vi "Measurement UI.vi"() -> ()   [LabVIEW 2021, in "ADC_ACMeasurement.lvlib"]
uses:
  adc_acMeasurement.lvlib
panel:
  in  "MeasGraphs":T1(tab)
  out "FreqDomainGraph":cluster{"x0":dbl, "dx":dbl, "magnitude":dbl[]}(graph) caption="AC"
  out "TimeDomainGraph":waveform(dbl)(graph) caption="AC"
  out "ENOB":dbl
  out "SFDR":dbl
  out "SINAD":dbl
  out "THD":dbl
  out "SNR":dbl
  out "Calculated amplitude":dbl
  out "Calculated frequency":dbl
  out "Channel name":string
  out "Time domain":dbl[](array[numeric])
  out "dt":dbl
  out "t0":dbl
  out "Spectrum":dbl[](array[numeric])
  out "df":dbl
  out "f0":dbl
  in  "Analog source resource name":string
  in  "Digital capture resource name":string
  out "MeasTable":string[][](table)
  in  "Digital capture":string="Digital capture"
  in  "Analog source":string="Analog source"
  in  "MeasSettingsOptions":i32(listbox)
  in  "MeasSettings":bool
  in  "Digital capture samples":u32=800000 caption="NUMBER OF SAMPLES"
  in  "Input channel":i32 caption="INPUT CHANNEL" min=0 max=100 step=1
  in  "Full scale range":dbl=10.0 caption="FULL SCALE RANGE" format="%#_6pV"
  in  "Digital capture sample rate":dbl=800000.0 caption="SAMPLE RATE" format="%#_6pS/s"
  in  "Amplitude":dbl=-1.0 caption="AMPLITUDE" format="%#_6pdB"
  in  "Frequency":dbl=1000.0 caption="FREQUENCY" format="%#_6pHz"
  in  "DSGResourceName":tag caption="RESOURCE NAME"
  in  "DPIResourceName":refnum<k15> caption="RESOURCE NAME"
  in  "ADCparameters":string="ADC parameters"
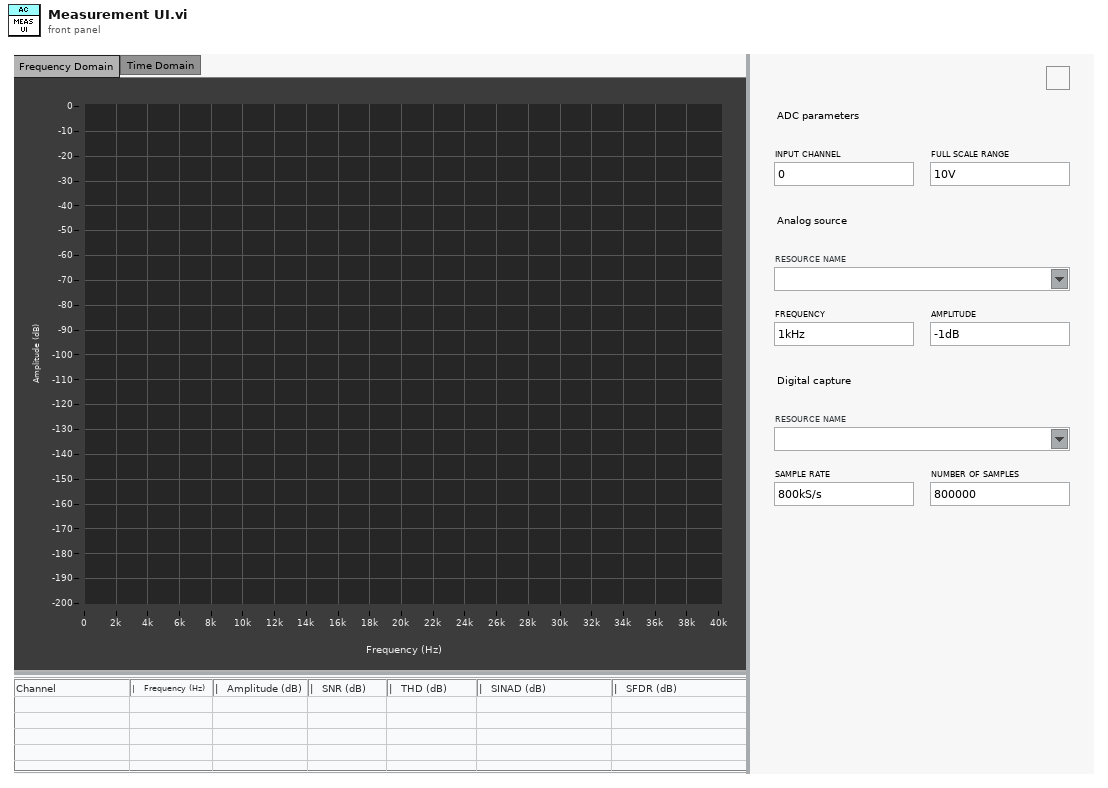
[diagram p1: front panel]
types:
  T1 = enum32{"Frequency Domain", "Time Domain", "Hidden Controls"}
  T2 = enum16{"open", "replace", "create", "open or create", "replace or create", "replace or create with confirmation"}
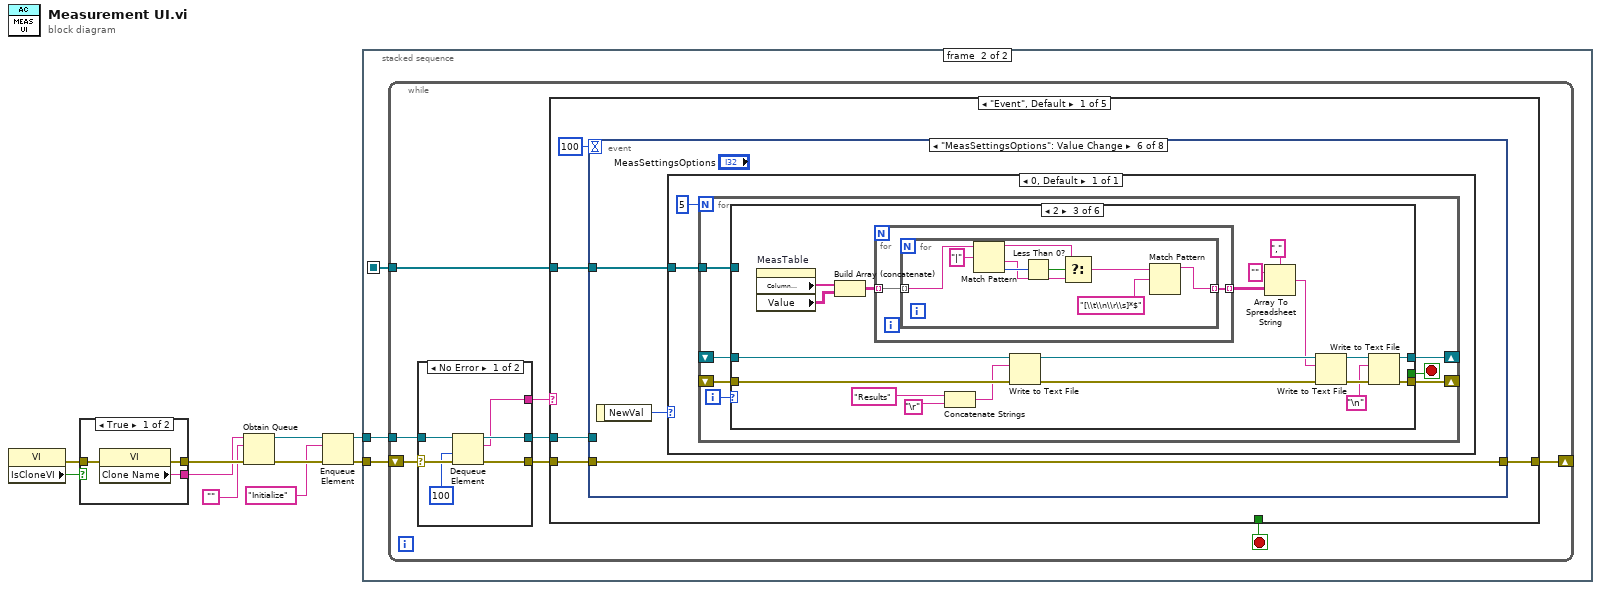
[diagram p0: block diagram]
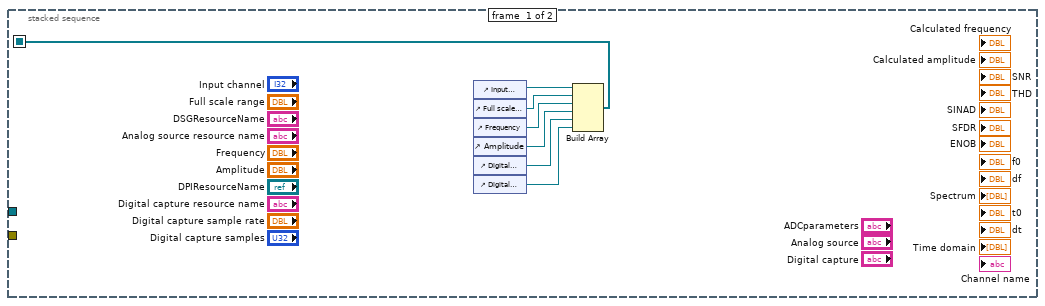
[diagram p2: hidden frame]
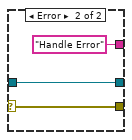
[diagram p3: hidden frame]
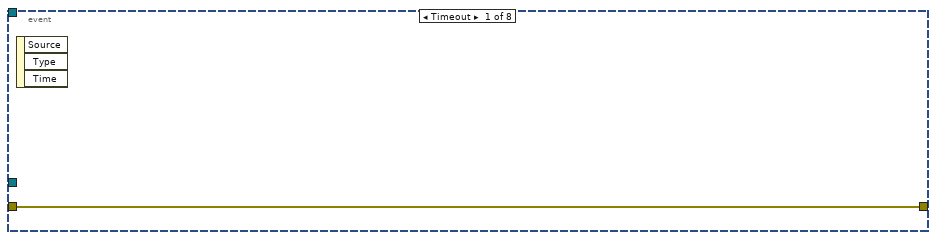
[diagram p4: hidden frame]
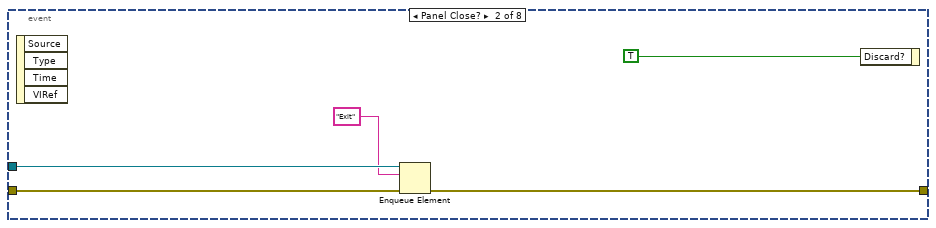
[diagram p5: hidden frame]
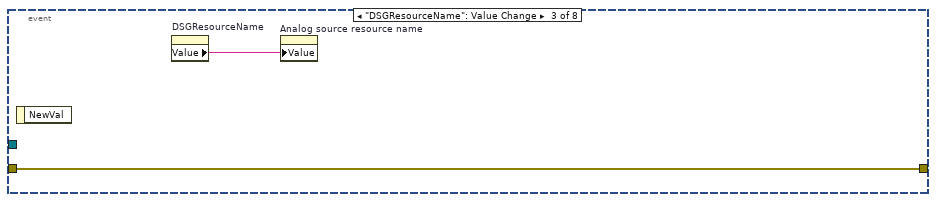
[diagram p6: hidden frame]
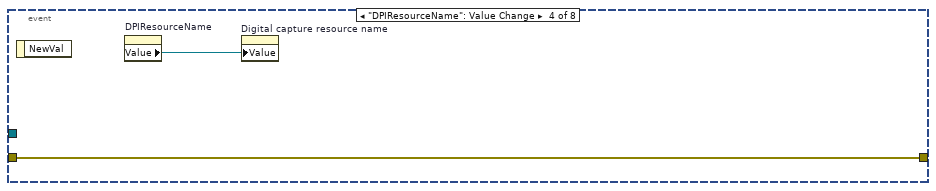
[diagram p7: hidden frame]
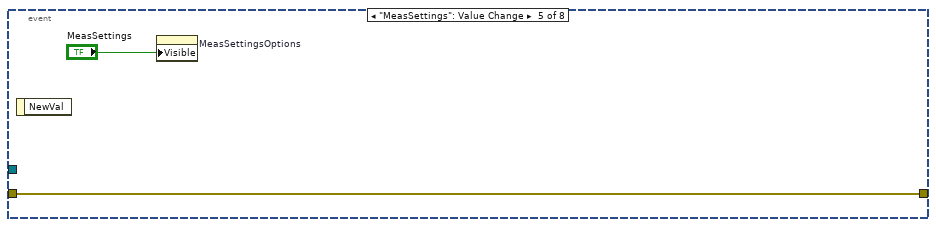
[diagram p8: hidden frame]
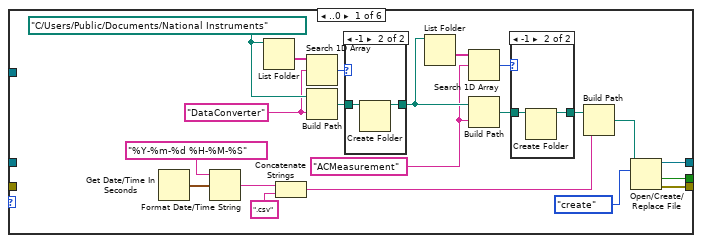
[diagram p9: hidden frame]
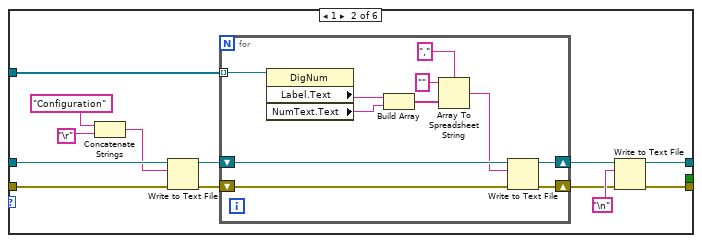
[diagram p12: hidden frame]
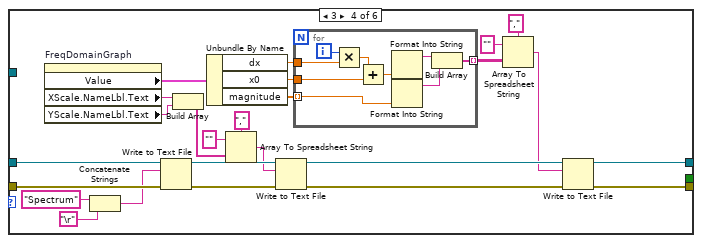
[diagram p13: hidden frame]
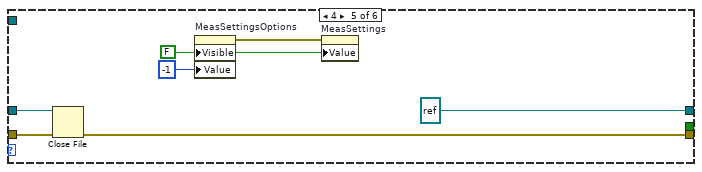
[diagram p14: hidden frame]
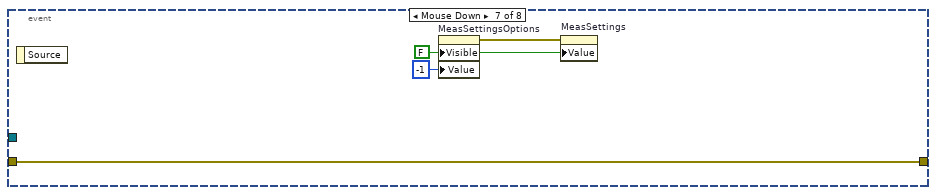
[diagram p16: hidden frame]
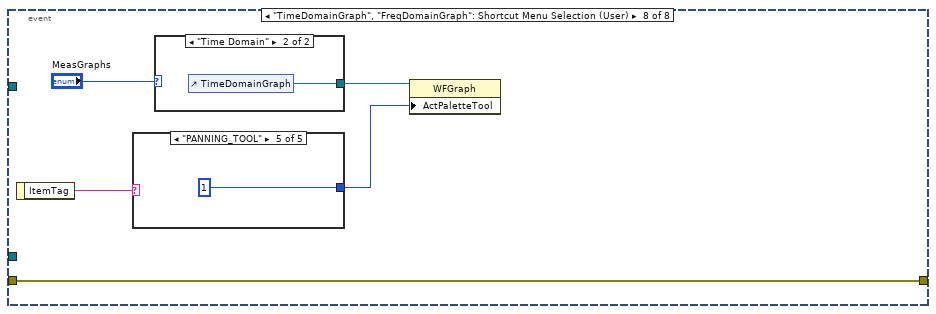
[diagram p17: hidden frame]
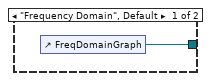
[diagram p18: hidden frame]
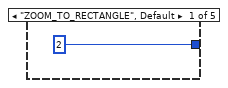
[diagram p19: hidden frame]
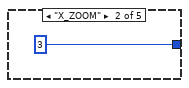
[diagram p20: hidden frame]
diagram:
  n1 = property class="VI"() -> (error out=w1:errorcluster, "IsCloneVI"=w2:bool)  [unwired: 2 in, 1 out]
  n2 = case shown="True" w2 {
    tunnel: [w13 w16] -> w10
    tunnel: [w12 w15] -> w9
    tunnel: w1 -> [w11 w14]
    frame True {
      n3 = property class="VI"(error in=w11) -> (error out=w13:errorcluster, "Clone Name"=w12:string)  [unwired: 1 in, 1 out]
    }
    frame False {
      n4 = property class="VI"(error in=w14) -> (error out=w16:errorcluster, "Name"=w15:string)  [unwired: 1 in, 1 out]
    }
  }
  n5 = Obtain Queue(name (unnamed)=w9, element data type="", error in (no error)=w10) -> (queue out=w6:refnum<queue>, error out=w8:errorcluster)  [unwired: 2 in, 1 out]
  n6 = Enqueue Element(queue=w6, element="Initialize", error in (no error)=w8) -> (queue out=w5:refnum<queue>, error out=w7:errorcluster)  [unwired: 1 in, 1 out]
  n7 = stacked-sequence {
    seq-local: [w17 _] -> [_ w24]
    tunnel: w7 -> [_ w26]
    tunnel: w5 -> [_ w25]
    frame #0 {
      n8 = control-ref of="Input channel"() -> (w23:refnum<vi>)
      n9 = control-ref of="Full scale range"() -> (w22:refnum<vi>)
      n10 = control-ref of="Frequency"() -> (w21:refnum<vi>)
      n11 = control-ref of="Amplitude"() -> (w20:refnum<vi>)
      n12 = control-ref of="Digital capture sample rate"() -> (w19:refnum<vi>)
      n13 = control-ref of="Digital capture samples"() -> (w18:refnum<vi>)
      n14 = Build Array(w23, w22, w21, w20, w19, w18) -> (w17:refnum<vi>[])
    }
    frame #1 {
      n15 = while {
        shift-right: [w29] -> _
        shift-left: w26 -> [w34]
        tunnel: w25 -> [w32]
        tunnel: w24 -> [w27]
        stop <- w28 stop-if-true
        n16 = case shown="No Error" w34 {
          selector: w34 -> [w40 w43]
          tunnel: [w39 w43] -> w33
          tunnel: w32 -> [w38 w42]
          tunnel: [w37 w42] -> w31
          tunnel: [w36 "Handle Error"] -> w30
          frame No Error {
            n17 = Dequeue Element(queue=w38, timeout in ms (-1)=100, error in (no error)=w40) -> (queue out=w37:refnum<queue>, element=w36:string, error out=w39:errorcluster)  [unwired: 1 out]
          }
          frame Error {
          }
        }
        n18 = case shown="\"Event\", Default" w30 {
          tunnel: w33 -> [w47 w220 w247 w262 w263]
          tunnel: w31 -> [w45 _ _ w260 _]
          tunnel: [w48 w220 w247 w257 w263] -> w29
          tunnel: [_ _ _ TRUE _] -> w28
          tunnel: w27 -> [w44 _ _ _ _]
          frame "Event", Default {
            n19 = event shown="[5] \"MeasSettingsOptions\": Value Change" {
              selector: _ -> [_ _ _ _ _ _ _ _]
              dyn-events: _ -> [_ _ _ _ _ _ _ _]
              timeout: 100 -> [_ _ _ _ _ _ _ _]
              tunnel: [w49 w52 w56 w57 w60 w62 w199 w205] -> w48
              tunnel: w47 -> [w49 w53 w56 w57 w60 w62 w199 w205]
              tunnel: w45 -> [_ w51 _ _ _ _ _ _]
              tunnel: w44 -> [_ _ _ _ _ w61 _ _]
              event Timeout {
                n20 = event-data() -> ()  [unwired: 1 in, 3 out]
              }
              event Panel Close? {
                n21 = event-data() -> ()  [unwired: 1 in, 4 out]
                n22 = Enqueue Element(queue=w51, element="Exit", error in (no error)=w53) -> (error out=w52:errorcluster)  [unwired: 1 in, 2 out]
                n23 = event-data("Discard?"=TRUE) -> ()  [unwired: 1 in, 1 out]
              }
              event "DSGResourceName": Value Change {
                n24 = event-data() -> ()  [unwired: 1 in, 1 out]
                n25 = property on="DSGResourceName" class="DAQmxName"() -> ("Value"=w55:string)  [unwired: 2 in, 2 out]
                n26 = property on="Analog source resource name" class="Str"("Value"=w55) -> ()  [unwired: 2 in, 2 out]
              }
              event "DPIResourceName": Value Change {
                n27 = event-data() -> ()  [unwired: 1 in, 1 out]
                n28 = property on="DPIResourceName" class="IVIName"() -> ("Value"=w58:refnum<k15>)  [unwired: 2 in, 2 out]
                n29 = property on="Digital capture resource name" class="Str"("Value"=w58) -> ()  [unwired: 2 in, 2 out]
              }
              event "MeasSettings": Value Change {
                n30 = event-data() -> ()  [unwired: 1 in, 1 out]
                n31 = property on="MeasSettingsOptions" class="LstBox (strict)"("Visible"="MeasSettings") -> ()  [unwired: 2 in, 2 out]
              }
              event "MeasSettingsOptions": Value Change {
                n32 = event-data() -> ("NewVal"=w63:i32)  [unwired: 1 in]
                n33 = case shown="0, Default" w63 {
                  tunnel: w61 -> [w64]
                  frame 0, Default {
                    n34 = for {
                      N: 5 -> [_]
                      shift-right: [w70] -> _
                      shift-left: _ -> [w69]
                      shift-right: [w68] -> _
                      shift-left: _ -> [w67]
                      tunnel: w64 -> [w66]
                      i -> [w72]
                      stop <- w71 stop-if-true
                      n35 = case shown="2" w72 {
                        tunnel: [w86 _ _ _ _ _] -> w71
                        tunnel: [w92 w102 w129 w164 refnum<file> refnum ("refnum out") w196] -> w70
                        tunnel: w69 -> [_ w110 w142 w178 w194 w196]
                        tunnel: [w85 w100 w128 w163 w192 w195] -> w68
                        tunnel: w67 -> [_ w108 w141 w177 w191 w195]
                        tunnel: w66 -> [_ w112 _ _ _ _]
                        frame ..0 {
                          w81 = "ACMeasurement" ("prompt")
                          w88 = "DataConverter" ("prompt")
                          w91 = path "C:/Users/Public/Documents/National Instruments" ("base path")
                          n36 = Get Date/Time In Seconds() -> (seconds since 1Jan1904=w78:timestamp)
                          n37 = Format Date/Time String(time format string (%c)="%Y-%m-%d %H-%M-%S", seconds (now)=w78) -> (date/time string=w77:string)  [unwired: 1 in]
                          n38 = List Folder(path=w91) -> (folder names=w89:string[])  [unwired: 3 in, 3 out]
                          n39 = Concatenate Strings(w77, ".csv" ("string")) -> (w74:string)
                          n40 = Search 1D Array(1D array=w89, element=w88) -> (index of element=w87:i32)  [unwired: 1 in]
                          n41 = Build Path(base path=w91, name or relative path=w88) -> (appended path=w90:path)
                          n42 = case shown="-1" w87 {
                            tunnel: w90 -> [w97 w99]
                            tunnel: [w97 w98] -> w82
                            frame Default {
                            }
                            frame -1 {
                              n43 = Create Folder(path (use dialog)=w99) -> (created path=w98:path)  [unwired: 2 in, 2 out]
                            }
                          }
                          n44 = List Folder(path=w82) -> (folder names=w84:string[])  [unwired: 3 in, 3 out]
                          n45 = Search 1D Array(1D array=w84, element=w81) -> (index of element=w83:i32)  [unwired: 1 in]
                          n46 = Build Path(base path=w82, name or relative path=w81) -> (appended path=w80:path)
                          n47 = case shown="-1" w83 {
                            tunnel: w80 -> [w94 w96]
                            tunnel: [w94 w95] -> w75
                            frame Default {
                            }
                            frame -1 {
                              n48 = Create Folder(path (use dialog)=w96) -> (created path=w95:path)  [unwired: 2 in, 2 out]
                            }
                          }
                          n49 = Build Path(base path=w75, name or relative path=w74) -> (appended path=w73:path)
                          n50 = Open/Create/Replace File(file path (use dialog)=w73, operation (0:open)=T2."create") -> (refnum out=w92:refnum<file>, cancelled=w86:bool, error out=w85:errorcluster)  [unwired: 4 in]
                        }
                        frame 1 {
                          n51 = Concatenate Strings("Configuration" ("format string"), "\r") -> (w105:string)
                          n52 = Write to Text File(file (use dialog)=w110, text=w105, error in=w108) -> (refnum out=w111:refnum<file>, error out=w109:errorcluster)  [unwired: 1 in, 1 out]
                          n53 = for {
                            tunnel: w112 -> [w123] mode=indexing
                            shift-right: [w114] -> w103
                            shift-left: w111 -> [w117]
                            shift-right: [w113] -> w101
                            shift-left: w109 -> [w116]
                            n54 = property class="DigNum"(reference=w123) -> ("Label.Text"=w122:string, "NumText.Text"=w121:string)  [unwired: 1 in, 2 out]
                            n55 = Build Array(w122, w121) -> (w120:string[])
                            n56 = Array To Spreadsheet String(delimiter (Tab)=",", array=w120, 3:"" ("format string")) -> (spreadsheet string=w115:string)
                            n57 = Write to Text File(file (use dialog)=w117, text=w115, error in=w116) -> (refnum out=w114:refnum<file>, error out=w113:errorcluster)  [unwired: 1 in, 1 out]
                          }
                          n58 = Write to Text File(file (use dialog)=w103, text="\n", error in=w101) -> (refnum out=w102:refnum<file>, error out=w100:errorcluster)  [unwired: 1 in, 1 out]
                        }
                        frame 2 {
                          n59 = property on="MeasTable" class="Tbl (strict)"() -> ("Column Headers[]"=w139:string[], "Value"=w138:string[][])  [unwired: 2 in, 2 out]
                          n60 = Build Array (concatenate)(w139, w138) -> (w137:string[][])
                          n61 = for {
                            tunnel: w137 -> [w144] mode=indexing
                            tunnel: [w143] -> w136 mode=indexing
                            n62 = for {
                              tunnel: w144 -> [w146] mode=indexing
                              tunnel: [w145] -> w143 mode=indexing
                              n63 = Match Pattern(string=w146, regular expression="|") -> (before substring=w150:string, after substring=w149:string, offset past match=w152:i32)  [unwired: 1 in, 1 out]
                              n64 = Less Than 0?(x=w152) -> (x < 0?=w151:bool)
                              n65 = Select(t=w150, s=w151, f=w149) -> (s? t:f=w148:string)
                              n66 = Match Pattern(string=w148, regular expression="[\\t\\n\\r\\s]*$") -> (before substring=w145:string)  [unwired: 1 in, 3 out]
                            }
                          }
                          n67 = Concatenate Strings("Results" ("element"), "\r") -> (w124:string)
                          n68 = Write to Text File(file (use dialog)=w142, text=w124, error in=w141) -> (refnum out=w140:refnum<file>, error out=w132:errorcluster)  [unwired: 1 in, 1 out]
                          n69 = Array To Spreadsheet String(delimiter (Tab)=",", array=w136, 3:"" ("format string")) -> (spreadsheet string=w133:string)
                          n70 = Write to Text File(file (use dialog)=w140, text=w133, error in=w132) -> (refnum out=w131:refnum<file>, error out=w130:errorcluster)  [unwired: 1 in, 1 out]
                          n71 = Write to Text File(file (use dialog)=w131, text="\n", error in=w130) -> (refnum out=w129:refnum<file>, error out=w128:errorcluster)  [unwired: 1 in, 1 out]
                        }
                        frame 3 {
                          n72 = property on="FreqDomainGraph" class="WFGraph (strict)"() -> ("Value"=w156:cluster{"x0":dbl, "dx":dbl, "magnitude":dbl[]}, "XScale.NameLbl.Text"=w174:string, "YScale.NameLbl.Text"=w173:string)  [unwired: 2 in, 2 out]
                          n73 = Concatenate Strings("Spectrum" ("string"), "\r") -> (w175:string)
                          n74 = Write to Text File(file (use dialog)=w178, text=w175, error in=w177) -> (refnum out=w169:refnum<file>, error out=w168:errorcluster)  [unwired: 1 in, 1 out]
                          n75 = Build Array(w174, w173) -> (w172:string[])
                          n76 = Unbundle By Name(w156) -> ("dx"=w158:dbl, "x0"=w159:dbl, "magnitude"=w157:dbl[])
                          n77 = Array To Spreadsheet String(delimiter (Tab)=",", array=w172, 3:"" ("format string")) -> (spreadsheet string=w167:string)
                          n78 = Write to Text File(file (use dialog)=w169, text=w167, error in=w168) -> (refnum out=w166:refnum<file>, error out=w165:errorcluster)  [unwired: 1 in, 1 out]
                          n79 = for {
                            tunnel: w157 -> [w182] mode=indexing
                            tunnel: w158 -> [w186]
                            tunnel: w159 -> [w184]
                            tunnel: [w179] -> w160 mode=indexing
                            i -> [w187]
                            n80 = Multiply(x=w187, y=w186) -> (x*y=w185:dbl)
                            n81 = Add(x=w185, y=w184) -> (x+y=w183:dbl)
                            n82 = Format Into String(w183) -> (resulting string=w180:string)  [unwired: 3 in, 1 out]
                            n83 = Format Into String(w182) -> (resulting string=w181:string)  [unwired: 3 in, 1 out]
                            n84 = Build Array(w180, w181) -> (w179:string[])
                          }
                          n85 = Array To Spreadsheet String(delimiter (Tab)=",", array=w160, 3:"" ("format string")) -> (spreadsheet string=w155:string)
                          n86 = Write to Text File(file (use dialog)=w166, text=w155, error in=w165) -> (refnum out=w164:refnum<file>, error out=w163:errorcluster)  [unwired: 1 in, 1 out]
                        }
                        frame 4 {
                          w189 = FALSE ("Visible")
                          n87 = Close File(refnum=w194, error in=w191) -> (error out=w192:errorcluster)  [unwired: 1 out]
                          n88 = property on="MeasSettingsOptions" class="LstBox (strict)"("Visible"=w189, "Value"=-1 ("MeasSettingsOptions")) -> (error out=w190:errorcluster)  [unwired: 2 in, 1 out]
                          n89 = property on="MeasSettings" class="Bool (strict)"(error in=w190, "Value"=w189) -> ()  [unwired: 1 in, 2 out]
                        }
                        frame Default {
                        }
                      }
                    }
                  }
                }
              }
              event Mouse Down {
                w197 = FALSE ("Visible")
                n90 = event-data() -> ()  [unwired: 1 in, 1 out]
                n91 = property on="MeasSettingsOptions" class="LstBox (strict)"("Visible"=w197, "Value"=-1 ("MeasSettingsOptions")) -> (error out=w198:errorcluster)  [unwired: 2 in, 1 out]
                n92 = property on="MeasSettings" class="Bool (strict)"(error in=w198, "Value"=w197) -> ()  [unwired: 1 in, 2 out]
              }
              event "TimeDomainGraph", "FreqDomainGraph": Shortcut Menu Selection (User) {
                n93 = event-data() -> ("ItemTag"=w204:string)  [unwired: 1 in]
                n94 = case shown="\"PANNING_TOOL\"" w204 {
                  tunnel: [2 ("Palette:Active Tool") 3 ("Palette:Active Tool") 4 ("Palette:Active Tool") 5 ("Palette:Active Tool") 1 ("Palette:Active Tool")] -> w201
                  frame "ZOOM_TO_RECTANGLE", Default {
                  }
                  frame "X_ZOOM" {
                  }
                  frame "Y_ZOOM" {
                  }
                  frame "ZOOM_TO_FIT" {
                  }
                  frame "PANNING_TOOL" {
                  }
                }
                n95 = case shown="\"Time Domain\"" "MeasGraphs" {
                  tunnel: [w206 w207] -> w202
                  frame "Frequency Domain", Default {
                    n96 = control-ref of="FreqDomainGraph"() -> (w206:refnum<vi>)
                  }
                  frame "Time Domain" {
                    n97 = control-ref of="TimeDomainGraph"() -> (w207:refnum<vi>)
                  }
                }
                n98 = property class="WFGraph"(reference=w202, "ActPaletteTool"=w201) -> ()  [unwired: 1 in, 2 out]
              }
            }
          }
          frame "Initialize" {
            w214 = 2 ("Palette:Active Tool")
            w218 = string[] ["Export data"] ("Item Names")
            w219 = "<Select Device>"
            n99 = property on="DSGResourceName" class="DAQmxName"("Value"=w219) -> ()  [unwired: 2 in, 2 out]
            n100 = property on="DPIResourceName" class="IVIName"("Value"=w219) -> ()  [unwired: 2 in, 2 out]
            n101 = property on="MeasGraphs" class="TabCtl (strict)"("Value"=T1."Frequency Domain" ("MeasGraphs")) -> ()  [unwired: 2 in, 2 out]
            n102 = property on="MeasSettingsOptions" class="LstBox (strict)"("Item Names"=w218, "Value"=-1 ("MeasSettingsOptions"), "Visible"=FALSE, "Disabled Items"=i32[] []) -> ()  [unwired: 2 in, 2 out]
            n103 = property on="TimeDomainGraph" class="WFGraph (strict)"("ActPaletteTool"=w214) -> ()  [unwired: 2 in, 2 out]
            n104 = for {
              tunnel: w218 -> [_] mode=indexing
              i -> [w222]
              n105 = property on="MeasSettingsOptions" class="LstBox (strict)"("Active Row"=w222, "Cell Height"=30 ("Active Row:Cell Height")) -> ()  [unwired: 2 in, 2 out]
            }
            n106 = property on="FreqDomainGraph" class="WFGraph (strict)"("ActPaletteTool"=w214) -> ()  [unwired: 2 in, 2 out]
          }
          frame "Post UI Update" {
            w232 = "|   " ("initial string")
            # "This case will be triggered, after framework updates the User interface with result values."
            n107 = local read "Spectrum"() -> (w225:dbl[])
            n108 = local read "Time domain"() -> (w244:dbl[])
            n109 = local read "df"() -> (w223:dbl)
            n110 = local read "Calculated amplitude"() -> (w241:dbl)
            n111 = local read "f0"() -> (w224:dbl)
            n112 = local read "Calculated frequency"() -> (w242:dbl)
            n113 = local read "dt"() -> (w245:dbl)
            n114 = local read "SINAD"() -> (w238:dbl)
            n115 = local read "ENOB"() -> (w236:dbl)
            n116 = Bundle By Name("dt"=w245, "Y"=w244) -> (→"TimeDomainGraph":waveform(dbl))  [unwired: 1 in]
            n117 = Bundle("f0"=w224, "df"=w223, "Spectrum"=w225) -> (→"FreqDomainGraph":cluster{"f0":dbl, "df":dbl, "Spectrum":dbl[]})  [unwired: 1 in]
            n118 = local read "SFDR"() -> (w237:dbl)
            n119 = local read "THD"() -> (w239:dbl)
            n120 = local read "SNR"() -> (w240:dbl)
            n121 = Build Array(w242, w241) -> (w235:dbl[])
            n122 = Build Array(w240, w239, w238, w237, w236) -> (w233:dbl[])
            n123 = local read "Channel name"() -> (w226:string)
            n124 = for {
              tunnel: w235 -> [w252] mode=indexing
              tunnel: w232 -> [w253]
              tunnel: "%.3f" ("initial string") -> [w254]
              tunnel: [w255] -> w230 mode=indexing
              n125 = Format Into String(format string=w254, initial string=w253, w252) -> (resulting string=w255:string)  [unwired: 1 in, 1 out]
            }
            n126 = for {
              tunnel: w233 -> [w248] mode=indexing
              tunnel: w232 -> [w249]
              tunnel: "%5.1f" ("initial string") -> [w250]
              tunnel: [w251] -> w229 mode=indexing
              n127 = Format Into String(format string=w250, initial string=w249, w248) -> (resulting string=w251:string)  [unwired: 1 in, 1 out]
            }
            n128 = Build Array (concatenate)(w226, w230, w229) -> (w228:string[])
            n129 = Build Array(w228) -> (→"MeasTable":string[][])
          }
          frame "Exit" {
            # "This case is triggered to close the User Interface from framework"
            n130 = Flush Queue(queue=w260, error in (no error)=w262) -> (queue out=w259:refnum<queue>, error out=w258:errorcluster)  [unwired: 1 out]
            n131 = Release Queue(queue=w259, force destroy? (F)=TRUE, error in (no error)=w258) -> (error out=w257:errorcluster)  [unwired: 2 out]
          }
          frame "Handle Error" {
          }
        }
      }
    }
  }
